vi "Agilent 2000 3000 X-Series Acquire Digital Voltmeter.vi"() -> ()   [LabVIEW 2015]
doc: "This example shows how to acquire digital voltmeter."
uses:
  Agilent 2000 3000 X-Series.lvlib
panel:
  out "5-digit Frequency":dbl
  out "3-digit DVM":dbl
  in  "VISA resource name":refnum<visa-resource-name>
  # "(c) 2011-2023 National Instruments.  ALL RIGHTS RESERVED."
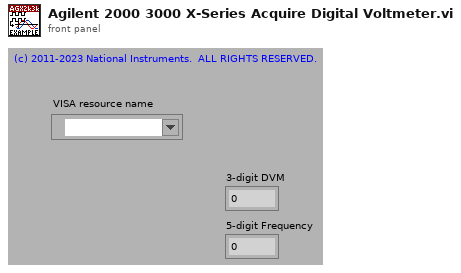
[diagram p1: front panel]
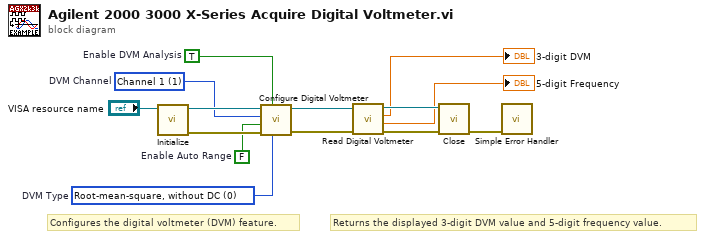
[diagram p0: block diagram]
diagram:
  w7 = 0 items=["Root-mean-square, without DC", "DC Value", "Root-mean-square", "Frequency Counter"]  # DVM Type
  w8 = TRUE  # Enable DVM Analysis
  w9 = FALSE  # Enable Auto Range
  w10 = 1 items=["Channel 1"=1, "Channel 2"=2, "Channel 3"=3, "Channel 4"=4]  # DVM Channel
  # "Returns the displayed 3-digit DVM value and 5-digit frequency value."
  # "Configures the digital voltmeter (DVM) feature."
  n1 = call "Initialize.vi"("VISA resource name"="VISA resource name") -> ("error out"=w12:errorcluster, "VISA resource name out"=w11:refnum<visa-resource-name>)  [unwired: 4 in, 5 out]
  n2 = call "Configure Digital Voltmeter.vi"("DVM Type (0: Root-mean-square, without DC)"=w7, "Enable DVM Analysis (F: Disable)"=w8, "error in (no error)"=w12, "Auto Range (F: Disable)"=w9, "DVM Channel (1: Channel 1)"=w10, "VISA resource name"=w11) -> ("error out"=w5:errorcluster, "VISA resource name out"=w6:refnum<visa-resource-name>)  [unwired: 4 out]
  n3 = call "Read Digital Voltmeter.vi"("error in (no error)"=w5, "VISA resource name"=w6) -> ("error out"=w3:errorcluster, "5-digit Frequency"=→"5-digit Frequency":dbl, "3-digit DVM"=→"3-digit DVM":dbl, "VISA resource name out"=w4:refnum<visa-resource-name>)  [unwired: 6 out]
  n4 = call "Close.vi"("error in (no error)"=w3, "VISA resource name"=w4) -> ("error out"=w13:errorcluster)  [unwired: 9 out]
  n5 = call <vilib>:"Simple Error Handler.vi"("error in (no error)"=w13) -> ()  [unwired: 1 in, 8 out]
